vi "Get_Mid_value.vi"(10 "Data array":sgl[][](array[numeric])) -> (2 "Output":dbl[](array[numeric]))   [LabVIEW 2019]
uses:
  <vilib>/Analysis/NI_AALBase.lvlib
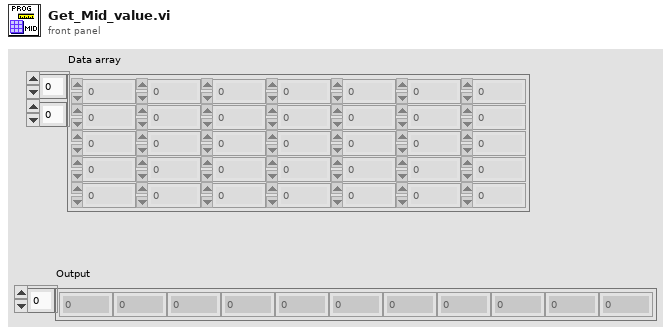
[diagram p1: front panel]
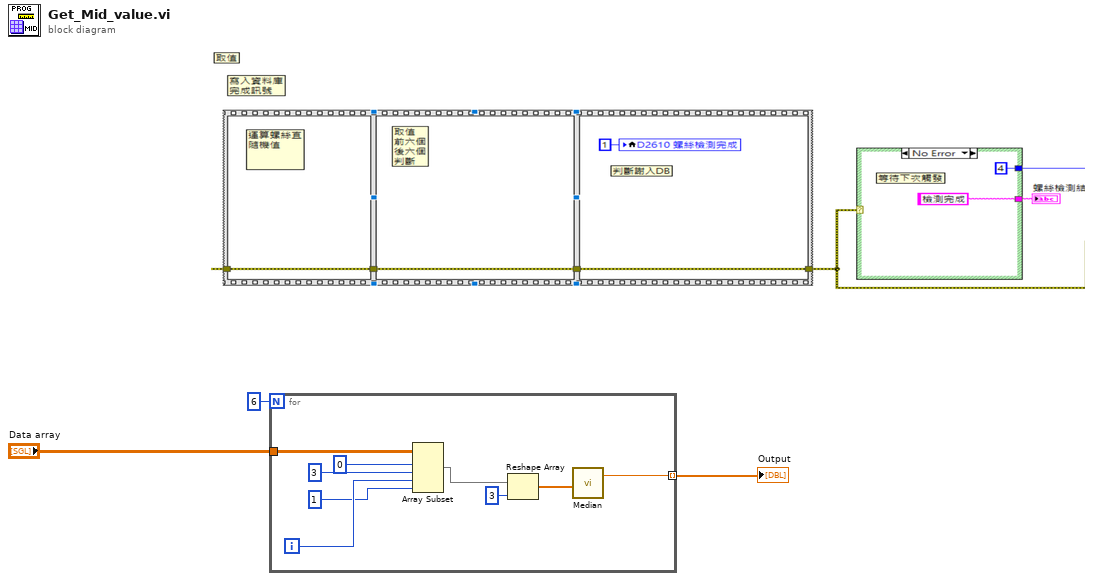
[diagram p0: block diagram]
diagram:
  n1 = for {
    N: 6 -> [_]
    tunnel: "Data array" -> [w8]
    tunnel: [w4] -> w1 mode=indexing
    i -> [w12]
    n2 = Array Subset(array=w8, index (row)=0 ("index"), length (row)=3 ("length"), index (col)=w12, length (col)=1 ("length")) -> (w7:sgl[][])
    n3 = Reshape Array(w7, 3 ("dimension size")) -> (w5:sgl[])
    n4 = call <vilib>:"Median.vi"("X"=w5) -> ("median"=w4:dbl)  [unwired: 1 out]
  }
  "Output" <- w1
